vi "Read Sensitivity(x).vi"(8 "error in (no error)":errorcluster, 11 "Joysticks in":refnum<class "Joysticks.lvclass">) -> (0 "error out":errorcluster, 2 "Sensitivity(x)":dbl, 3 "Joysticks out":refnum<class "Joysticks.lvclass">)   [LabVIEW 2019, in "Joysticks.lvlib" / "Joysticks.lvclass"]
uses:
  Joysticks.lvclass
  Joysticks.lvclass/Joysticks.ctl
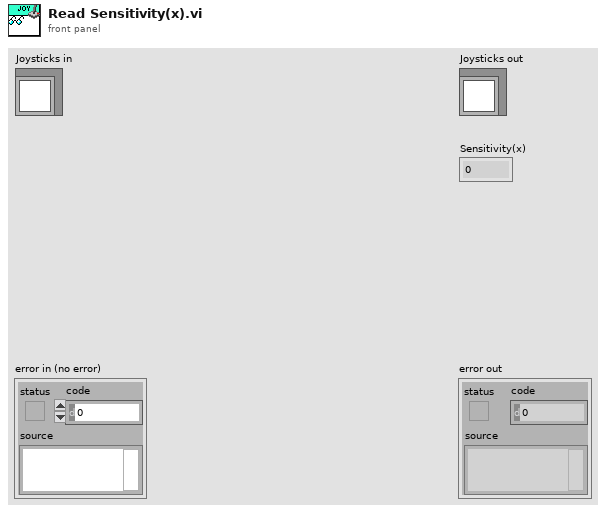
[diagram p1: front panel]
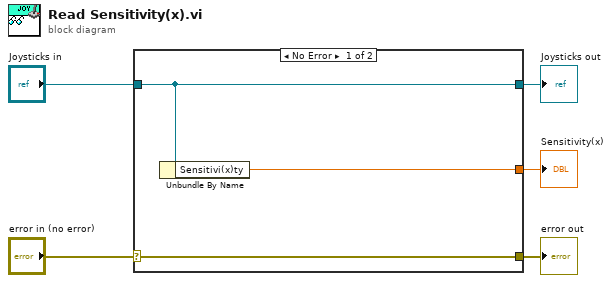
[diagram p0: block diagram]
diagram:
  n1 = case shown="No Error" "error in (no error)" {
    selector: "error in (no error)" -> [w8 w9]
    tunnel: [w8 w9] -> w4
    tunnel: [w7 w10] -> w2
    tunnel: "Joysticks in" -> [w7 w10]
    tunnel: [w6 _] -> w1
    frame No Error {
      n2 = Unbundle By Name(w7) -> ("Sensitivi(x)ty"=w6:dbl)
    }
    frame Error {
    }
  }
  "error out" <- w4
  "Joysticks out" <- w2
  "Sensitivity(x)" <- w1
